vi "close.vi"(8 "error in (no error)":errorcluster, 11 "AnalogOutput in":refnum<class "AnalogOutput.lvclass">) -> (0 "error out":errorcluster)   [LabVIEW 2009, in "Hardware.lvlib" / "Channels.lvlib" / "AnalogOutput.lvclass"]
doc: "Closes the analog output device."
uses:
  AnalogOutput.lvclass
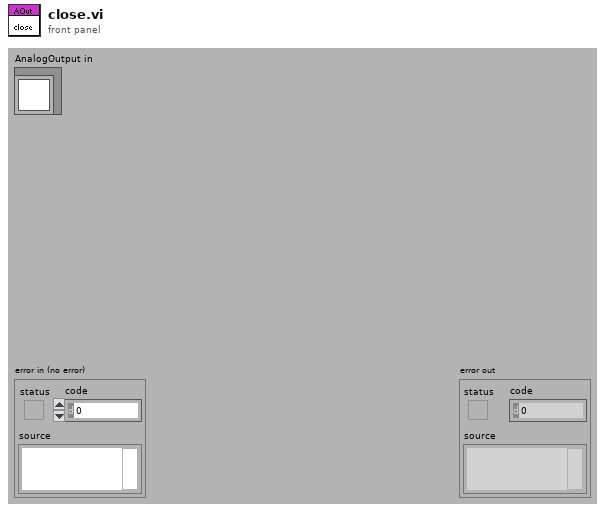
[diagram p1: front panel]
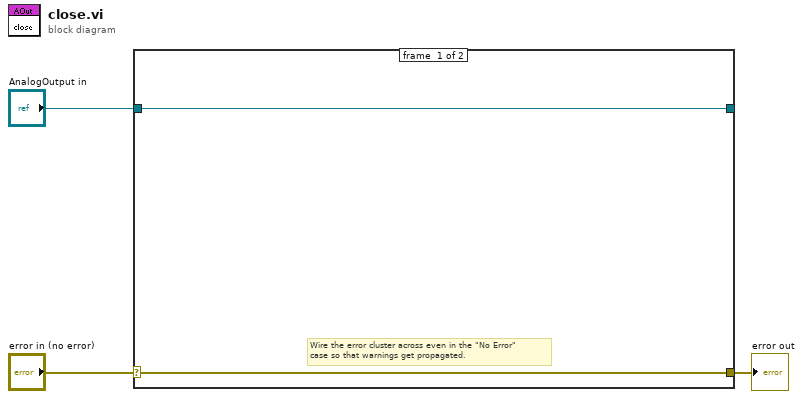
[diagram p0: block diagram]
diagram:
  n1 = case shown="No Error" "error in (no error)" {
    selector: "error in (no error)" -> [w4 w7]
    tunnel: [w4 w7] -> w2
    tunnel: [w5 w6] -> _
    tunnel: "AnalogOutput in" -> [w5 w6]
    frame #0 {
      # "Wire the error cluster across even in the \"No Error\"\ncase so that warnings get propagated."
    }
    frame #1 {
    }
  }
  "error out" <- w2
